vi "L03P03.vi"() -> ()   [LabVIEW 2020]
uses:
  <vilib>/MakerHub/LINX/Public/Peripherals/Digital/Digital Read 1 Chan.vi
  <vilib>/MakerHub/LINX/Public/Peripherals/Digital/Digital Write 1 Chan.vi
  <vilib>/MakerHub/LINX/Public/Peripherals/Digital/Digital Read N Chans.vi
  <vilib>/MakerHub/LINX/Public/Peripherals/Digital/Digital Write N Chans.vi
  <vilib>/MakerHub/LINX/Private/Local IO/LinxDigitalRead.vi
  <vilib>/MakerHub/LINX/Public/Utilities/Check Channel.vi
  <vilib>/MakerHub/LINX/Private/Local IO/LinxDigitalWrite.vi
  <vilib>/MakerHub/LINX/Public/Utilities/Open Serial.vi
  <vilib>/MakerHub/LINX/Private/Utilties/Generate Error.vi
  <vilib>/MakerHub/LINX/LMH-LINX.lvlib
panel:
  in  "Invert Behaviour":bool
  in  "stop":bool
  out "Number of Tilts vs Time":i32(graph)
  out "Tilted":bool
  # "Adam Sokacz\n400177446\n3CC3\nLab 3"
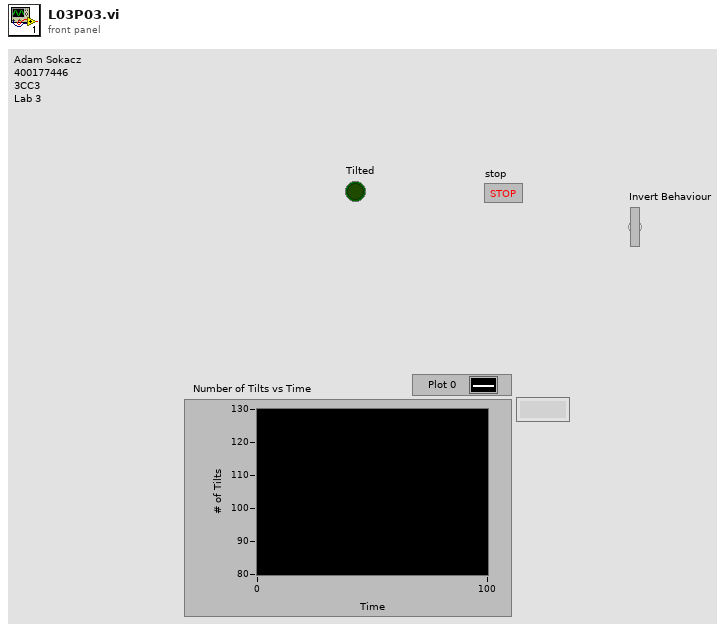
[diagram p1: front panel]
types:
  T1 = typedef "LMH-LINX.lvlib/LINX Ref.ctl" = cluster{"IO":T2, "Interface":T3, "LINX Device Config":T4}
  T2 = typedef "LMH-LINX.lvlib/Platform.ctl" = enum16{"Remote", "Local"}
  T3 = typedef "LMH-LINX.lvlib/Interface.ctl" = enum16{"Serial", "TCP"}
  T4 = typedef "LMH-LINX.lvlib/Device.lvlib/LINX Device Config.ctl" = cluster{"Interface":T3, "COM Port":refnum<visa-resource-name>, "TCP Configuration":T5, "Device Family":u8, "Device ID":u8, "Device Name":string, "TCP Ref":refnum<k5>, "Channels":T6}
  T5 = typedef "LMH-LINX.lvlib/Device.lvlib/TCP Config.ctl" = cluster{"IP Address":string, "Port":u16}
  T6 = typedef "LMH-LINX.lvlib/Channels.ctl" = cluster{"DI":u8[], "DO":u8[], "AI":u8[], "AO":u8[], "PWM":u8[], "QE":u8[], "UART":u8[], "I2C 2":u8[], "SPI":u8[], "CAN":u8[], "Servo":u8[], "AI Ref (V)":dbl, "AI Resolution (Bits)":u8, "AO Ref (V)":dbl, "AO Resolution (Bits)":u8}
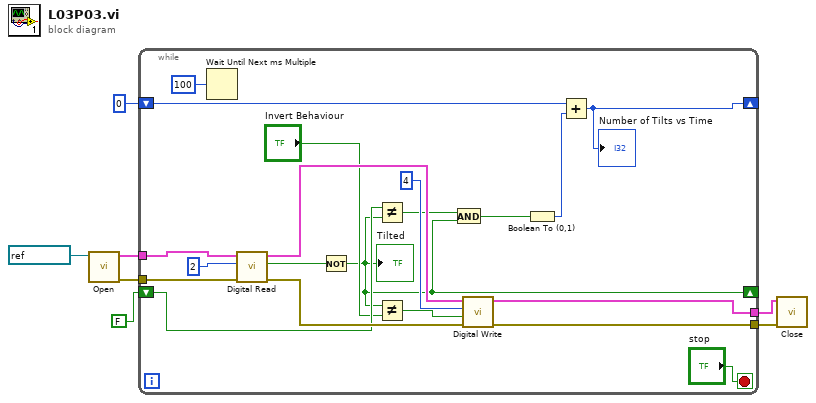
[diagram p0: block diagram]
diagram:
  n1 = call-poly <vilib>:"Open.vi"("Serial Port"=refnum<visa-resource-name> "COM8") -> ("Error Out"=w5:errorcluster, "LINX Resource"=w6:T1)  [unwired: 8 in, 1 out]
  n2 = while {
    tunnel: w6 -> [w22]
    tunnel: w5 -> [w26]
    tunnel: [w24] -> w4
    tunnel: [w20] -> w3
    shift-right: [w13] -> _
    shift-left: 0 -> [w14]
    shift-right: [w8] -> _
    shift-left: FALSE -> [w18]
    stop <- "stop" stop-if-true
    n3 = Wait Until Next ms Multiple(millisecond multiple=u32 100) -> ()  [unwired: 1 out]
    n4 = call-poly <vilib>:"Digital Read.vi"("Error In"=w26, "DI Channel"=u8 2, "LINX Resource"=w22) -> ("Error Out"=w25:errorcluster, "DI Value"=w9:bool, "LINX Resource"=w21:T1)  [unwired: 6 in]
    n5 = Not(x=w9) -> (.not. x?=w8:bool)
    "Tilted" <- w8
    n6 = Not Equal?(x=w18, y=w8) -> (x != y?=w17:bool)
    n7 = Not Equal?(x=w8, y="Invert Behaviour") -> (x != y?=w10:bool)
    n8 = And(x=w17, y=w8) -> (x .and. y?=w16:bool)
    n9 = call-poly <vilib>:"Digital Write.vi"("Error In"=w25, "Output Value"=w10, "DO Channel"=u8 4, "LINX Resource"=w21) -> ("Error Out"=w24:errorcluster, "LINX Resource"=w20:T1)  [unwired: 6 in]
    n10 = Boolean To (0,1)(Boolean=w16) -> (0, 1=w15:i16)
    n11 = Add(x=w14, y=w15) -> (x+y=w13:i32)
    "Number of Tilts vs Time" <- w13
  }
  n12 = call <vilib>:"Close.vi"("Error In"=w4, "LINX Resource"=w3) -> ()  [unwired: 9 in, 1 out]
